vi "AdjustPreionTimings.vi"(1 "Input Trigger Data":T3) -> (0 "Output Trigger Data":T3)   [LabVIEW 2009]
uses:
  Ctrl_Signal.ctl
  Ctrl_Signal_Map.ctl
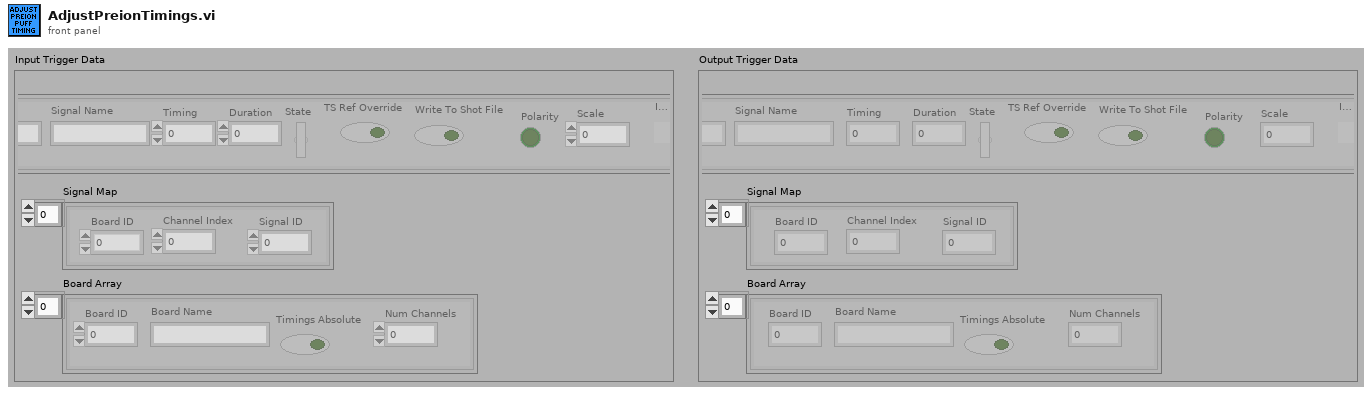
[diagram p1: front panel]
types:
  T1 = typedef "Ctrl_Signal.ctl" = cluster{"Signal Name":string, "Timing":dbl, "Duration":dbl, "State":bool, "TS Ref Override":bool, "Write To Shot File":bool, "Polarity":bool, "Signal ID":dbl, "Scale":dbl, "IsDelay":bool}
  T2 = typedef "Ctrl_Signal_Map.ctl" = cluster{"Channel Index":dbl, "Board ID":dbl, "Signal ID":dbl}
  T3 = cluster{"Signal Array":T1[], "Signal Map":T2[], "Board Array":cluster{"Board ID":dbl, "Board Name":string, "Timings Absolute":bool, "Num Channels":dbl}[]}
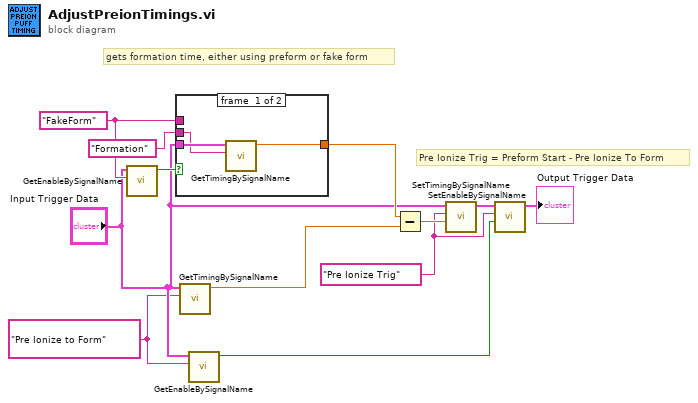
[diagram p0: block diagram]
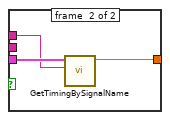
[diagram p2: hidden frame]
diagram:
  w10 = "FakeForm" ("Signal Name")
  w4 = "Pre Ionize Trig" ("Signal Name")
  w2 = "Pre Ionize to Form" ("Signal Name")
  # "gets formation time, either using preform or fake form"
  # "Pre Ionize Trig = Preform Start - Pre Ionize To Form"
  n1 = call "GetEnableBySignalName.vi"("Signal Name"=w10, "Trigger Data"="Input Trigger Data") -> ("Signal Enabled"=w11:bool)  [unwired: 9 in]
  n2 = case shown="False" w11 {
    tunnel: "Input Trigger Data" -> [w15 w18]
    tunnel: w10 -> [_ w17]
    tunnel: "Formation" ("Signal Name") -> [w14 _]
    tunnel: [w13 w16] -> w7
    frame #0 {
      n3 = call "GetTimingBySignalName.vi"("Signal Name"=w14, "Trigger Data"=w15) -> ("Timing"=w13:dbl)  [unwired: 9 in]
    }
    frame #1 {
      n4 = call "GetTimingBySignalName.vi"("Signal Name"=w17, "Trigger Data"=w18) -> ("Timing"=w16:dbl)  [unwired: 9 in]
    }
  }
  n5 = call "GetTimingBySignalName.vi"("Signal Name"=w2, "Trigger Data"="Input Trigger Data") -> ("Timing"=w8:dbl)  [unwired: 9 in]
  n6 = call "GetEnableBySignalName.vi"("Signal Name"=w2, "Trigger Data"="Input Trigger Data") -> ("Signal Enabled"=w1:bool)  [unwired: 9 in]
  n7 = Subtract(x=w7, y=w8) -> (x-y=w12:dbl)
  n8 = call "SetTimingBySignalName.vi"("Timing"=w12, "Signal Name"=w4, "Trigger Data Input"="Input Trigger Data") -> ("Trigger Data Output"=w6:T3)  [unwired: 8 in]
  n9 = call "SetEnableBySignalName.vi"("State"=w1, "Signal Name"=w4, "Trigger Data Input"=w6) -> ("Trigger Data Output"=→"Output Trigger Data":T3)  [unwired: 8 in]
